vi "Easy Generate XML.vi"(8 "error in (no error)":errorcluster, 10 "LabVIEW Data":variant) -> (0 "error out":errorcluster, 2 "XML String":string)   [LabVIEW 2013]
doc: "Converts <B>LabVIEW Data</B> to an XML string with the LabVIEW data names (labels) converted to XML item names and the LabVIEW data values converted to XML item values."
uses:
  Options API/Private/EasyXML Options - Data Cluster.ctl
  Options API/Private/EasyXML Options - Type Formatting Cluster.ctl
  Support/Type Defs/Formatting Data Type -- Enum.ctl
panel:
  # "JKI EasyXML Toolkit for LabVIEW\nhttp://jki.net/easyxml\nCopyright (C) 2007-2016, JKI <info@jki.net>\nALL RIGHTS RESERVED"
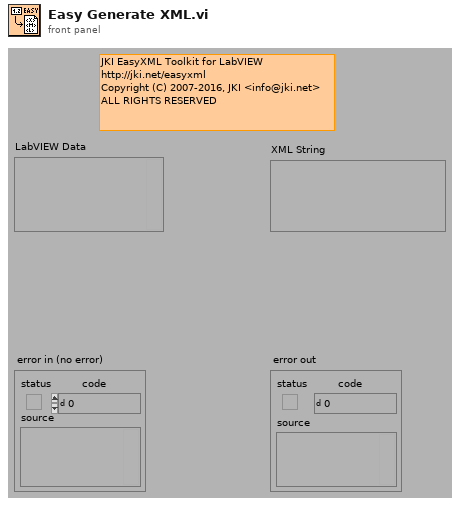
[diagram p1: front panel]
types:
  T1 = typedef "EasyXML Options - Data Cluster.ctl" = cluster{"Type Formatting":T2, "indentation spaces per level":i32}
  T2 = typedef "EasyXML Options - Type Formatting Cluster.ctl" = cluster{"Data Types":T3[], "Format Strings":string[]}
  T3 = typedef "Formatting Data Type -- Enum.ctl" = enum16{"<unknown>", "Cluster", "Array", "String", "Path", "Boolean", "Time Stamp", "Enum", "Numeric - EXT", "Numeric - DBL", "Numeric - SGL", "Numeric - I64", "Numeric - I32", "Numeric - I16", "Numeric - I8", "Numeric - U64", "Numeric - U32", "Numeric - U16", "Numeric - U8", "Numeric - CXT", "Numeric - CDB", "Numeric - CSG", "VISA Resource"}
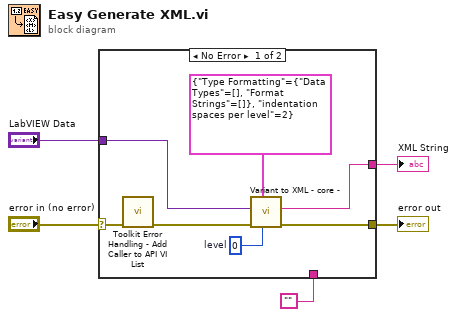
[diagram p0: block diagram]
diagram:
  n1 = case shown="No Error" "error in (no error)" {
    selector: "error in (no error)" -> [w7 w14]
    tunnel: [w12 w14] -> w4
    tunnel: "LabVIEW Data" -> [w10 _]
    tunnel: [w11 w13] -> w2
    tunnel: "" -> [_ w13]
    frame No Error {
      w8 = 0  # level
      n2 = call "Toolkit Error Handling - Add Caller to API VI List.vi"("error in"=w7) -> ("error out"=w6:errorcluster)  [unwired: 10 in]
      n3 = call "Variant to XML - core - .vi"("level"=w8, "Easy XML Options in"=T1 {"Type Formatting"={"Data Types"=[], "Format Strings"=[]}, "indentation spaces per level"=2}, "error in (no error)"=w6, "LabVIEW Data"=w10) -> ("error out"=w12:errorcluster, "XML String"=w11:string)  [unwired: 6 in]
    }
    frame Error {
    }
  }
  "error out" <- w4
  "XML String" <- w2
